vi "TA_Plot_Kinetics_2.vi"(0 "TA Data":T1={"DeltaA (mOD)"=array214x154[32956 elements], "Wavelength (nm)"=[410.0, 411.0, 413.0, 415.0, 416.0, 418.0, 420.0, 421.0, 423.0, 425.0, 426.0, 428.0, 430.0, 431.0, 433.0, 434.0, 436.0, 438.0, 439.0, 441.0, 443.0, 444.0, 446.0, 448.0, 449.0, 451.0, 453.0, 454.0, 456.0, 458.0, 459.0, 461.0, 462.0, 464.0, 466.0, 467.0, 469.0, 471.0, 472.0, 474.0, 476.0, 477.0, 479.0, 481.0, 482.0, 484.0, 485.0, 487.0, 489.0, 490.0, 492.0, 494.0, 495.0, 497.0, 499.0, 500.0, 502.0, 504.0, 505.0, 507.0, 508.0, 510.0, 512.0, 513.0, 515.0, 517.0, 518.0, 520.0, 522.0, 523.0, 525.0, 527.0, 528.0, 530.0, 531.0, 533.0, 535.0, 536.0, 538.0, 540.0, 541.0, 543.0, 545.0, 546.0, 548.0, 549.0, 551.0, 553.0, 554.0, 556.0, 558.0, 559.0, 561.0, 563.0, 564.0, 566.0, 568.0, 569.0, 571.0, 572.0, 574.0, 576.0, 577.0, 579.0, 581.0, 582.0, 584.0, 586.0, 587.0, 589.0, 590.0, 592.0, 594.0, 595.0, 597.0, 599.0, 600.0, 602.0, 604.0, 605.0, 607.0, 608.0, 610.0, 612.0, 613.0, 615.0, 617.0, 618.0, 620.0, 622.0, 623.0, 625.0, 626.0, 628.0, 630.0, 631.0, 633.0, 635.0, 636.0, 638.0, 639.0, 641.0, 643.0, 644.0, 646.0, 648.0, 649.0, 651.0, 653.0, 654.0, 656.0, 657.0, 659.0, 661.0, 662.0, 664.0, 666.0, 667.0, 669.0, 670.0, 672.0, 674.0, 675.0, 677.0, 679.0, 680.0, 682.0, 683.0, 685.0, 687.0, 688.0, 690.0, 692.0, 693.0, 695.0, 696.0, 698.0, 700.0, 701.0, 703.0, 705.0, 706.0, 708.0, 709.0, 711.0, 713.0, 714.0, 716.0, 718.0, 719.0, 721.0, 722.0, 724.0, 726.0, 727.0, 729.0, 731.0, 732.0, 734.0, 735.0, 737.0, 739.0, 740.0, 742.0, 744.0, 745.0, 747.0, 748.0, 750.0, 752.0, 753.0, 755.0, 757.0, 758.0], "Time (ps)"=[-8.0, -7.0, -6.0, -5.0, -4.0, -3.0, -2.0, -1.0, -0.0, -0.0, -0.0, -0.0, -0.0, -0.0, -0.0, -0.0, -0.0, -0.0, -0.0, -0.0, -0.0, -0.0, -0.0, -0.0, 0.0, 0.0, 0.0, 0.0, 0.0, 0.0, 0.0, 0.0, 0.0, 0.0, 0.0, 0.0, 0.0, 0.0, 0.0, 0.0, 0.0, 0.0, 0.0, 0.0, 1.0, 1.0, 1.0, 1.0, 1.0, 1.0, 1.0, 1.0, 1.0, 1.0, 1.0, 1.0, 2.0, 2.0, 2.0, 2.0, 2.0, 2.0, 3.0, 3.0, 3.0, 3.0, 3.0, 4.0, 4.0, 4.0, 4.0, 4.0, 5.0, 5.0, 5.0, 6.0, 6.0, 7.0, 7.0, 8.0, 8.0, 9.0, 9.0, 10.0, 11.0, 12.0, 13.0, 14.0, 15.0, 16.0, 17.0, 18.0, 19.0, 20.0, 22.0, 24.0, 26.0, 28.0, 30.0, 32.0, 34.0, 36.0, 38.0, 40.0, 42.0, 44.0, 46.0, 48.0, 50.0, 55.0, 60.0, 65.0, 70.0, 75.0, 80.0, 85.0, 90.0, 95.0, 100.0, 110.0, 120.0, 130.0, 140.0, 150.0, 160.0, 170.0, 180.0, 190.0, 200.0, 220.0, 240.0, 260.0, 280.0, 300.0, 320.0, 340.0, 360.0, 380.0, 400.0, 420.0, 440.0, 460.0, 480.0, 500.0, 550.0, 600.0, 650.0, 700.0, 750.0, 800.0, 850.0, 900.0, 950.0, 1000.0], "Size of DeltaA"=[214, 154], "Size of Wavelength"=214, "Size of Time"=154}) -> (7 "TA Kinetics":cluster{"Array":dbl[], "Array 2":dbl[]}[](graph))   [LabVIEW 2025]
uses:
  TA_DATA.ctl
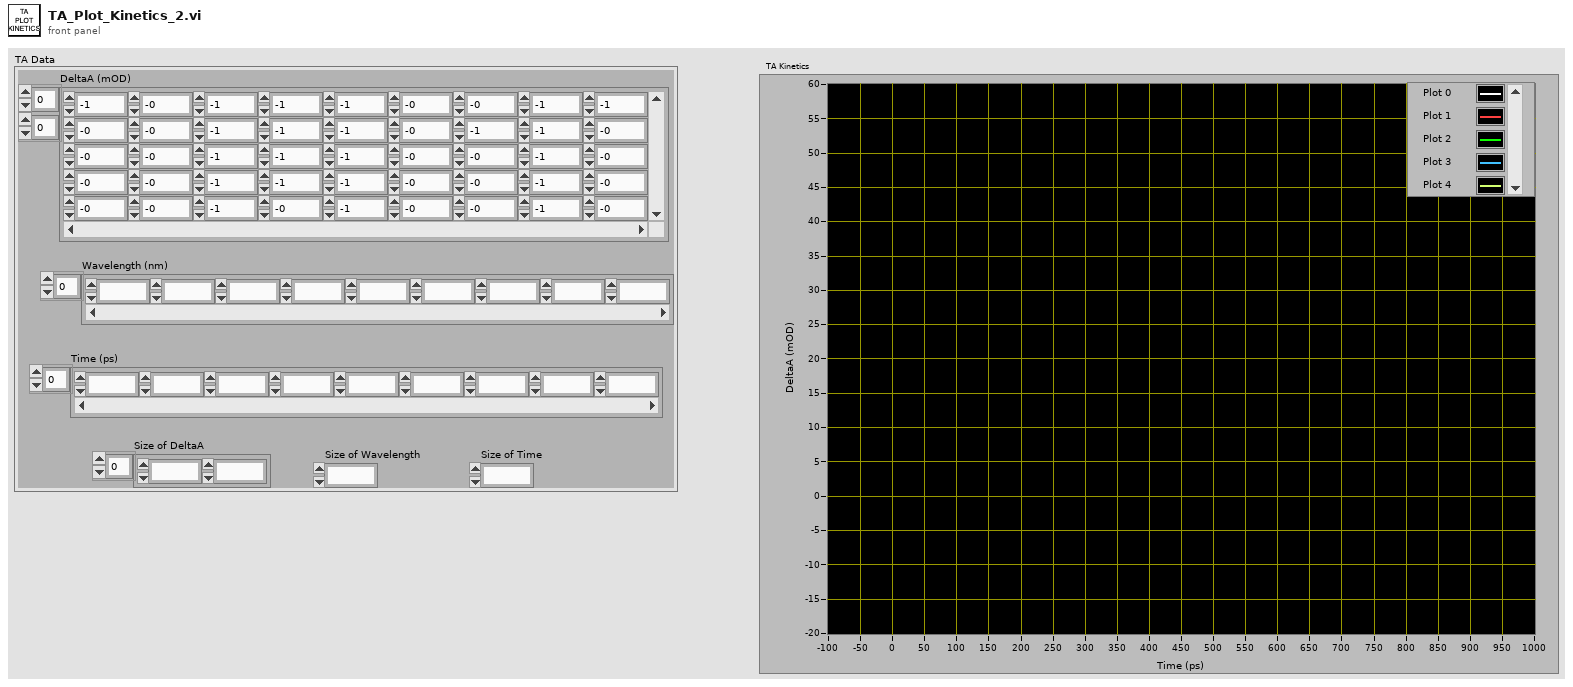
[diagram p1: front panel]
types:
  T1 = typedef "TA_DATA.ctl" = cluster{"DeltaA (mOD)":dbl[][], "Wavelength (nm)":dbl[], "Time (ps)":dbl[], "Size of DeltaA":i32[], "Size of Wavelength":i32, "Size of Time":i32}
  T2 = cluster{"Time (ps)":dbl[], "DeltaA (mOD)":dbl[]}[]
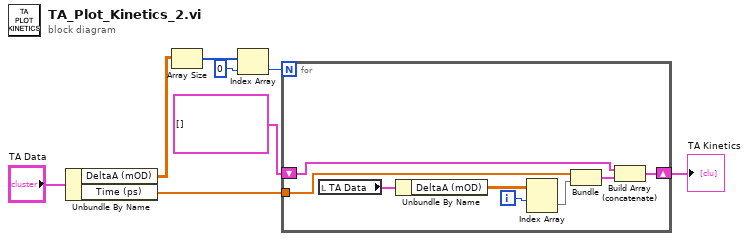
[diagram p0: block diagram]
diagram:
  n1 = Unbundle By Name("TA Data") -> ("DeltaA (mOD)"=w1:dbl[][], "Time (ps)"=w2:dbl[])
  n2 = Array Size(array=w1) -> (size(s)=w5:i32[])
  n3 = Index Array(array=w5, index=0) -> (element=w4:i32)
  n4 = for {
    N: w4 -> [_]
    tunnel: w2 -> [w16]
    shift-right: [w11] -> w8
    shift-left: cluster{"Array":dbl[], "Array 2":dbl[]}[] [] ("Array") -> [w13]
    i -> [w15]
    n5 = local read "TA Data"() -> (w10:T1)
    n6 = Unbundle By Name(w10) -> ("DeltaA (mOD)"=w9:dbl[][])
    n7 = Index Array(array=w9, index (row)=w15) -> (element=w14:dbl[])  [unwired: 1 in]
    n8 = Bundle("Time (ps)"=w16, "DeltaA (mOD)"=w14) -> (w12:cluster{"Time (ps)":dbl[], "DeltaA (mOD)":dbl[]})  [unwired: 1 in]
    n9 = Build Array (concatenate)(w13, w12) -> (w11:T2)
  }
  "TA Kinetics" <- w8
